vi "Teleop.vi"(10 "Match Info":T1={"Autonomous Elapsed Seconds"=0.0, "TeleOp Elapsed Seconds"=0.0, "Disabled Elapsed Seconds"=0.0, "Visited Autonomous"=FALSE, "Visited TeleOp"=FALSE, "Visited Disabled"=FALSE, "Autonomous Settings"={"Autonomous Style"=enum."Independent", "VI Refnum"=refnum}}, 11 "Call Context":T2) -> ()   [LabVIEW 2016]
doc: "This VI is called for each TeleOp packet received from the DS where the robot is not disabled. It is often used to read from the joysticks and update I/O or to update setpoints for timed control loops. It should complete and return within 20 milliseconds or it may miss DS packets."
uses:
  <vilib>/Rock Robotics/WPI/DriverStation/WPI_DriverStationDerivedRobotMode.ctl
  <vilib>/Rock Robotics/WPI/DriverStation/WPI_DriverStationMatch Info.ctl
  <vilib>/Rock Robotics/WPI/Relay/WPI_RelayValue.ctl
  <vilib>/Rock Robotics/WPI/Solenoid/WPI_SolenoidValue.ctl
  <vilib>/Rock Robotics/WPI/ThirdParty/CanMotor/TalonSRX/WPI_CANTalonSRX_BrakeOverride.ctl
  <vilib>/Rock Robotics/WPI/Utilities/WPI_GetSetVariantRefNum.vi
  <vilib>/Rock Robotics/Network Tables/NT Write Boolean Array.vi
  <vilib>/Rock Robotics/Network Tables/NT Write Numeric Array.vi
  <vilib>/Rock Robotics/Network Tables/NT Read Boolean.vi
  <vilib>/Rock Robotics/Network Tables/NT Read Number.vi
  <vilib>/Rock Robotics/Network Tables/NT Write Boolean.vi
  <vilib>/addons/control/pid/pid.llb/PID (DBL).vi
  <vilib>/Rock Robotics/WPI/Solenoid/WPI_SolenoidSetEnum.vi
  <vilib>/Rock Robotics/WPI/RobotDrive/WPI_RobotDriveArcadeDrive_Standard(NoSaturation).vi
  <vilib>/addons/control/pid/NI_PID_pid.lvlib
panel:
  out "percentRateLeft":dbl
  out "percentRateRight":dbl
  out "motorOutputInit":dbl
  out "motorOutputInit":dbl
  out "encRateLeft":dbl
  out "encRateRight":dbl
  out "outputLeft":dbl format="%.2f"
  out "outputRight":dbl format="%.2f"
  out "Sample Slider 0":dbl(slide) scale=0.0..5.0
  out "Sample Boolean 1":bool
  out "Sample Boolean 0":bool
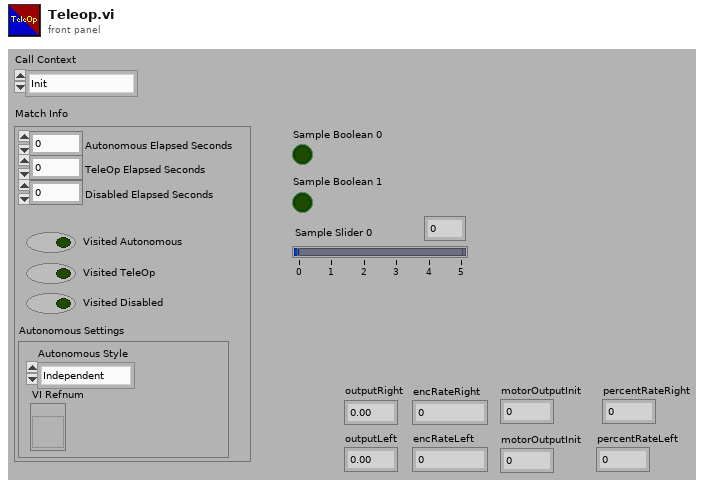
[diagram p1: front panel]
types:
  T1 = typedef "WPI_DriverStationMatch Info.ctl" = cluster{"Autonomous Elapsed Seconds":dbl, "TeleOp Elapsed Seconds":dbl, "Disabled Elapsed Seconds":dbl, "Visited Autonomous":bool, "Visited TeleOp":bool, "Visited Disabled":bool, "Autonomous Settings":cluster{"Autonomous Style":enum16{"Iterative", "Independent"}, "VI Refnum":refnum<vi>}}
  T2 = typedef "WPI_DriverStationDerivedRobotMode.ctl" = enum16{"Init", "Execute", "Stop"}
  T3 = cluster{"proportional gain (Kc)":dbl, "integral time (Ti, min)":dbl, "derivative time (Td, min)":dbl}
  T4 = typedef "WPI_CANTalonSRX_BrakeOverride.ctl" = enum8{"No Override", "Override to Coast", "Override to Brake"}
  T5 = typedef "WPI_SolenoidValue.ctl" = enum16{"Off", "On", "Forward", "Reverse"}
  T6 = typedef "WPI_RelayValue.ctl" = enum16{"Off", "On", "Forward", "Reverse"}
  T7 = typedef "WPI_JoystickDevRef.ctl" = cluster{"Device":T8}
  T8 = typedef "WPI_JoystickDeviceEnum.ctl" = enum16{"USB 0", "USB 1", "USB 2", "USB 3", "USB 4", "USB 5"}
  T9 = typedef "WPI_RobotDriveDevRef.ctl" = cluster{"DevStatus":errorcluster, "Motors[]":T10[], "Square Inputs":bool, "Max Output":dbl}
  T10 = typedef "WPI_MotorControlDeviceRef.ctl" = cluster{"DeviceStatus":errorcluster, "Type":T11, "PWM":cluster{"PWM Channel":T12, "DeadBand":T13}, "CAN":cluster{"Device Number":u8, "SetOutput VI Ref":variant, "GetOutput VI Ref":variant, "Enable VI Ref":variant, "Disable VI Ref":variant, "Data":variant}, "Invert":bool}
  T11 = typedef "WPI_MotorControlType.ctl" = enum16{"PWM", "CAN"}
  T12 = typedef "FPGA_DIOPWMChannel.ctl" = enum8{"PWM 0", "PWM 1", "PWM 2", "PWM 3", "PWM 4", "PWM 5", "PWM 6", "PWM 7", "PWM 8", "PWM 9", "PWM MXP 0", "PWM MXP 1", "PWM MXP 2", "PWM MXP 3", "PWM MXP 4", "PWM MXP 5", "PWM MXP 6", "PWM MXP 7", "PWM MXP 8", "PWM MXP 9", "Invalid"}
  T13 = typedef "WPI_PWMDeadband.ctl" = cluster{"Name":string, "maxPositivePwm":i32, "minPositivePwm":i32, "centerPwm":i32, "maxNegativePwm":i32, "minNegativePwm":i32, "angularRange":u16}
  T14 = typedef "WPI_RelayDevRef.ctl" = cluster{"DevStatus":errorcluster, "Relay Channel":T15, "Relay Direction":T16}
  T15 = typedef "FPGA_DIORelayChannel.ctl" = enum8{"Relay 0", "Relay 1", "Relay 2", "Relay 3", "Invalid"}
  T16 = typedef "WPI_RelayDirection.ctl" = enum16{"Both directions", "Forward only", "Reverse only"}
  T17 = typedef "WPI_SolenoidDevRef.ctl" = cluster{"DevStatus":errorcluster, "Pneumatics Control Module":u8, "Forward Solenoid Channel":T18, "Reverse Solenoid Channel":T18}
  T18 = typedef "WPI_SolenoidChannel.ctl" = enum8{"Solenoid 0", "Solenoid 1", "Solenoid 2", "Solenoid 3", "Solenoid 4", "Solenoid 5", "Solenoid 6", "Solenoid 7", "Invalid"}
  T19 = typedef "WPI_EncoderDevRef.ctl" = cluster{"DevStatus":errorcluster, "EncoderIndex":T20, "CounterIndex":T21, "DistancePerCount":dbl, "Decoding Type":T22}
  T20 = typedef "FPGA_EncoderIdx.ctl" = enum8{"Enc 0", "Enc 1", "Enc 2", "Enc 3", "Enc 4", "Enc 5", "Enc 6", "Enc 7", "Invalid"}
  T21 = typedef "FPGA_CounterCtrSystemIndex.ctl" = enum8{"Ctr 0", "Ctr 1", "Ctr 2", "Ctr 3", "Ctr 4", "Ctr 5", "Ctr 6", "Ctr 7", "Invalid"}
  T22 = typedef "WPI_EncoderType.ctl" = enum16{"1x", "2x", "4x"}
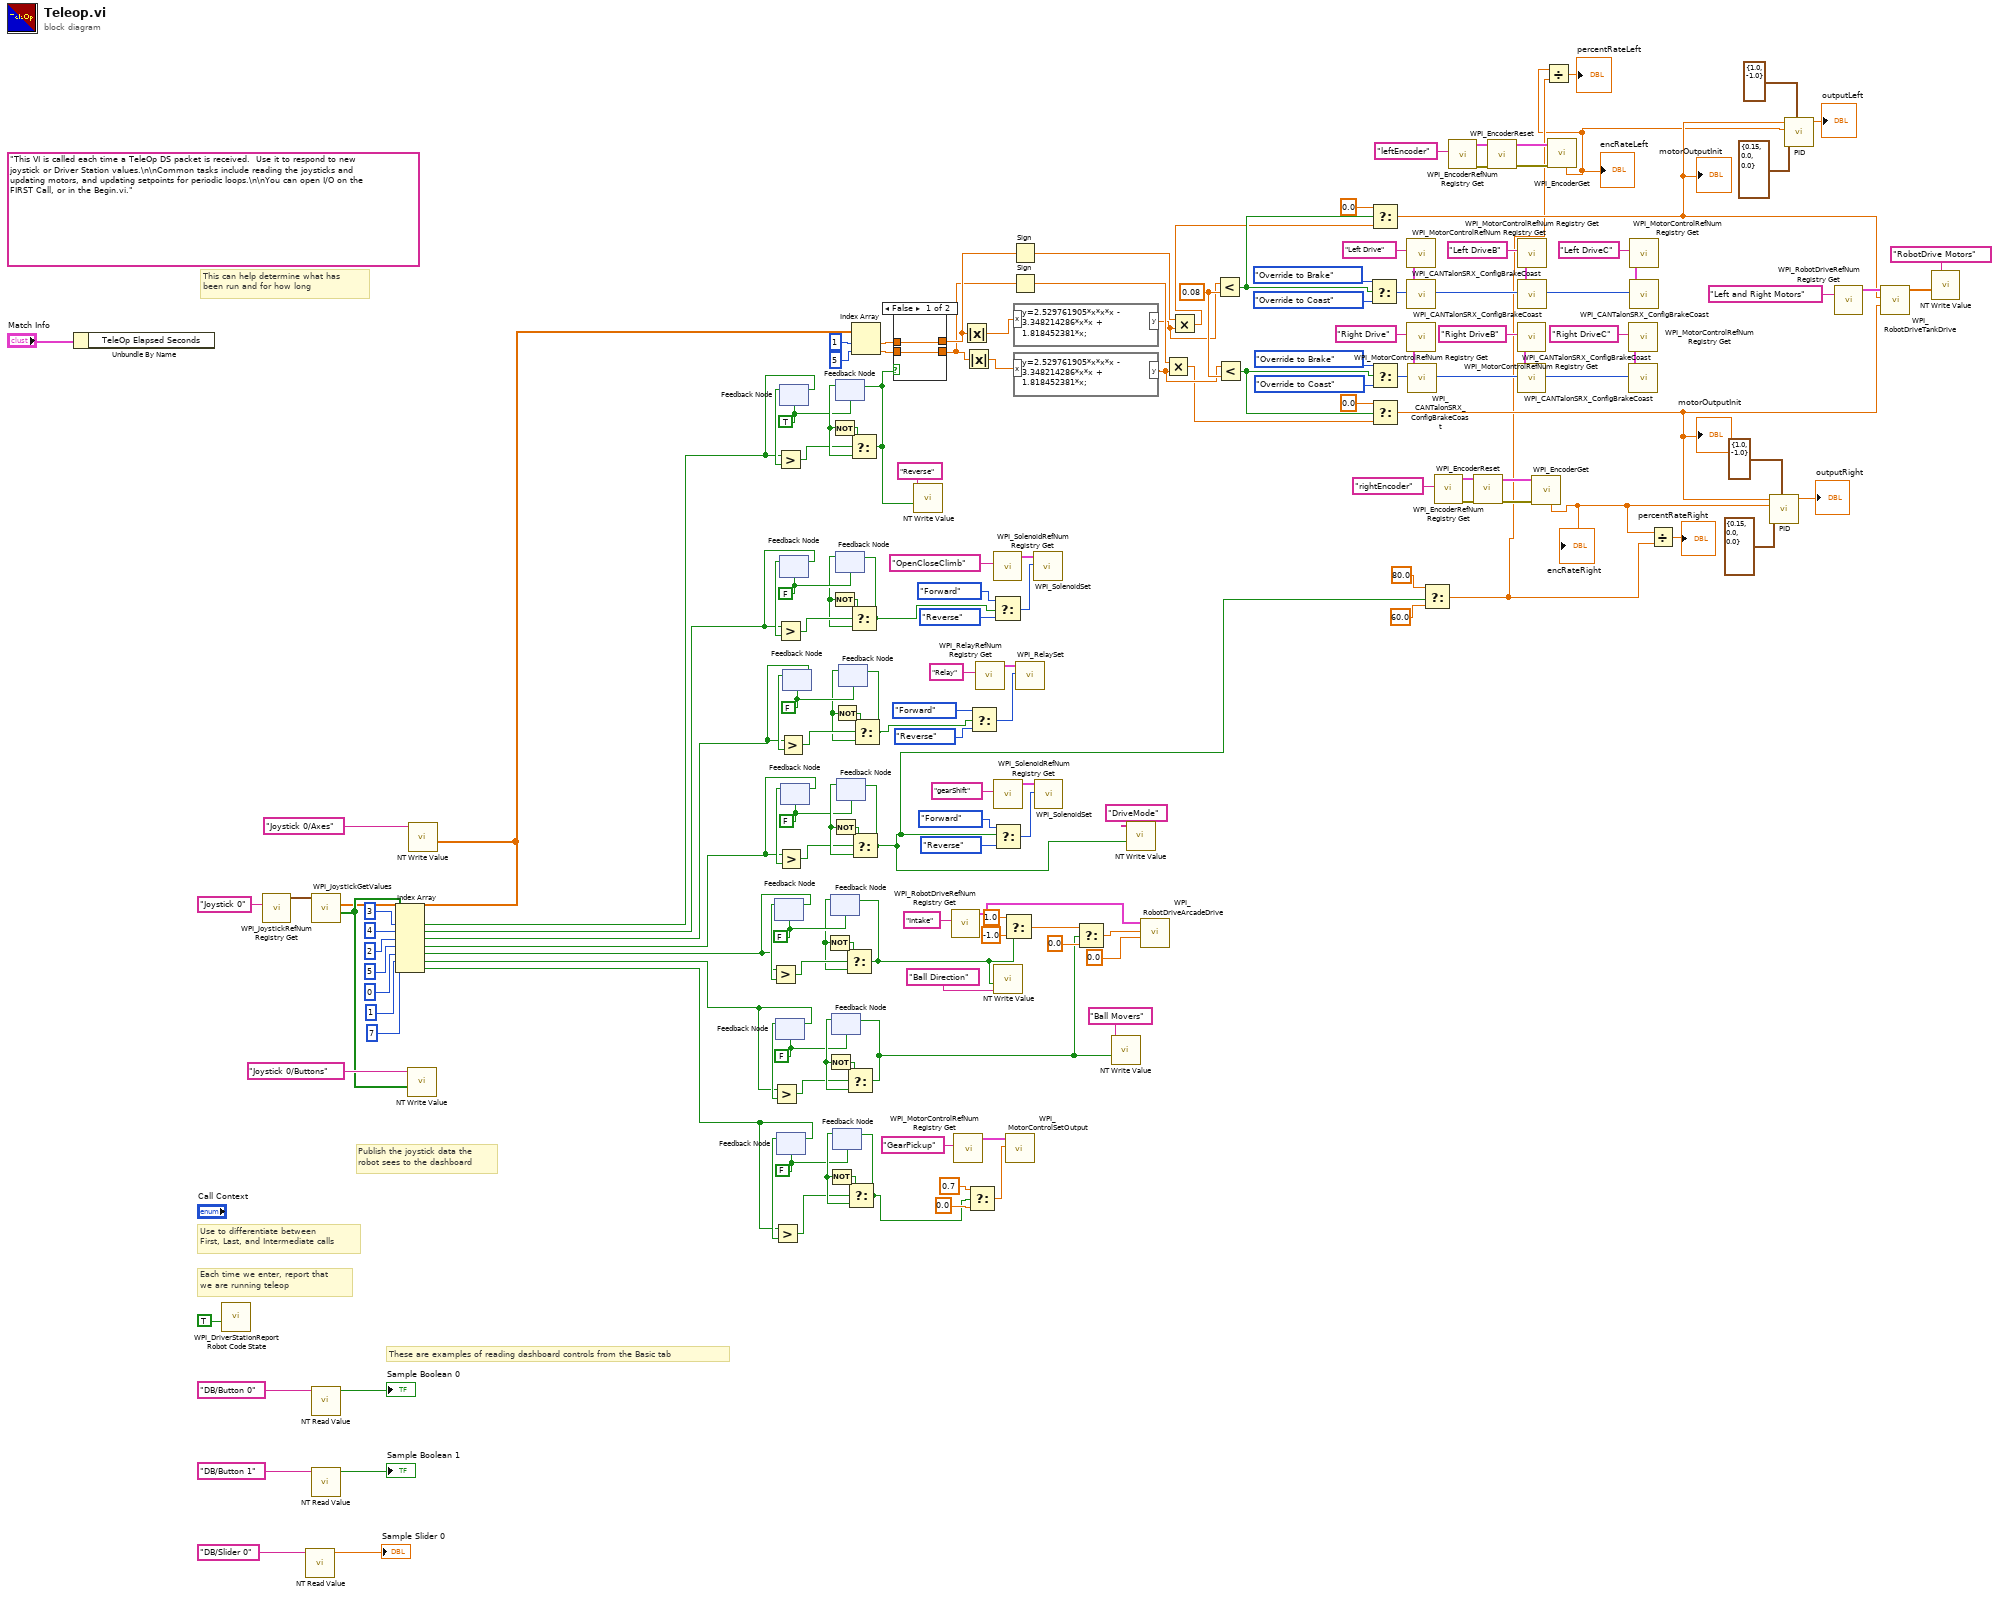
[diagram p0: block diagram]
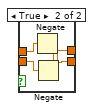
[diagram p2: hidden frame]
diagram:
  w45 = 0.08 ("y")
  w73 = TRUE ("Boolean")
  w102 = FALSE ("Boolean")
  w128 = FALSE ("Boolean")
  w133 = FALSE ("Boolean")
  w138 = FALSE ("Boolean")
  w143 = FALSE ("Boolean")
  w148 = FALSE ("Boolean")
  (unwired) "This VI is called each time a TeleOp DS packet is received.  Use it to respond to new joystick or Driver Station values.\n\nCommon tasks include reading the joysticks and updating motors, and updating setpoints for periodic loops.\n\nYou can open I/O on the FIRST Call, or in the Begin.vi."
  # "These are examples of reading dashboard controls from the Basic tab"
  # "Publish the joystick data the\nrobot sees to the dashboard"
  # "Each time we enter, report that\nwe are running teleop"
  # "Use to differentiate between\nFirst, Last, and Intermediate calls"
  # "This can help determine what has\nbeen run and for how long"
  n1 = Unbundle By Name("Match Info") -> ()  [unwired: 1 out]
  n2 = call <vilib>:"WPI_DriverStationReport Robot Code State.vi"("TeleOp"=TRUE ("Autonomous")) -> ()  [unwired: 10 in, 1 out]
  n3 = call <vilib>:"WPI_JoystickRefNum Registry Get.vi"("refnum name"="Joystick 0") -> ("JoystickDevRef"=w166:T7)  [unwired: 1 in, 9 out]
  n4 = call-poly <vilib>:"NT Read Value.vi"("Name"="DB/Slider 0" ("refnum name")) -> ("Numeric"=→"Sample Slider 0":dbl)  [unwired: 9 in, 1 out]
  n5 = call <vilib>:"WPI_JoystickGetValues.vi"("JoystickDevRef"=w166) -> ("Buttons"=w156:bool[], "Axes"=w67:dbl[])  [unwired: 6 in, 3 out]
  n6 = call-poly <vilib>:"NT Read Value.vi"("Name"="DB/Button 0" ("refnum name")) -> ("Boolean"=→"Sample Boolean 0":bool)  [unwired: 9 in, 1 out]
  n7 = call-poly <vilib>:"NT Read Value.vi"("Name"="DB/Button 1" ("refnum name")) -> ("Boolean"=→"Sample Boolean 1":bool)  [unwired: 9 in, 1 out]
  n8 = Index Array(array=w156, index #1=3 ("index"), index #2=4 ("index"), index #3=2 ("index"), index #4=5 ("index"), index #5=0 ("index"), index #6=1 ("index"), index #7=7 ("index")) -> (element #1=w66:bool, element #2=w65:bool, element #3=w64:bool, element #4=w63:bool, element #5=w62:bool, element #6=w61:bool, element #7=w60:bool)
  n9 = call-poly <vilib>:"NT Write Value.vi"("Boolean Array"=w156, "Name"="Joystick 0/Buttons") -> ()  [unwired: 9 in, 1 out]
  n10 = call-poly <vilib>:"NT Write Value.vi"("Numeric Array"=w67, "Name"="Joystick 0/Axes") -> ()  [unwired: 9 in, 1 out]
  n11 = feedback #1(w133) -> (w135:bool)
  n12 = Greater?(x=w62, y=w135) -> (0:w134:bool)
  n13 = feedback-in #1(w62) -> ()
  n14 = feedback #2(w102) -> (w100:bool)
  n15 = Greater?(x=w61, y=w100) -> (0:w101:bool)
  n16 = feedback-in #2(w61) -> ()
  n17 = feedback #3(w128) -> (w126:bool)
  n18 = Greater?(x=w60, y=w126) -> (0:w127:bool)
  n19 = feedback-in #3(w60) -> ()
  n20 = feedback #4(w73) -> (w71:bool)
  n21 = Greater?(x=w66, y=w71) -> (0:w72:bool)
  n22 = feedback-in #4(w66) -> ()
  n23 = feedback #5(w148) -> (w150:bool)
  n24 = Greater?(x=w65, y=w150) -> (0:w149:bool)
  n25 = feedback-in #5(w65) -> ()
  n26 = feedback #6(w138) -> (w136:bool)
  n27 = Greater?(x=w63, y=w136) -> (0:w137:bool)
  n28 = feedback-in #6(w63) -> ()
  n29 = feedback #7(w143) -> (w145:bool)
  n30 = Greater?(x=w64, y=w145) -> (0:w144:bool)
  n31 = feedback-in #7(w64) -> ()
  n32 = feedback #8(w133) -> (w132:bool)
  n33 = Not(x=w132) -> (.not. x?=w131:bool)
  n34 = feedback #9(w102) -> (w103:bool)
  n35 = Not(x=w103) -> (.not. x?=w104:bool)
  n36 = feedback #10(w128) -> (w129:bool)
  n37 = Not(x=w129) -> (.not. x?=w130:bool)
  n38 = feedback #11(w73) -> (w74:bool)
  n39 = Not(x=w74) -> (.not. x?=w75:bool)
  n40 = feedback #12(w148) -> (w147:bool)
  n41 = Not(x=w147) -> (.not. x?=w146:bool)
  n42 = feedback #13(w138) -> (w139:bool)
  n43 = Not(x=w139) -> (.not. x?=w140:bool)
  n44 = feedback #14(w143) -> (w142:bool)
  n45 = Not(x=w142) -> (.not. x?=w141:bool)
  n46 = Select(t=w131, s=w134, f=w132) -> (s? t:f=w84:bool)
  n47 = feedback-in #8(w84) -> ()
  n48 = Select(t=w104, s=w101, f=w103) -> (s? t:f=w85:bool)
  n49 = feedback-in #9(w85) -> ()
  n50 = Select(t=w130, s=w127, f=w129) -> (s? t:f=w89:bool)
  n51 = feedback-in #10(w89) -> ()
  n52 = Select(t=w75, s=w72, f=w74) -> (s? t:f=w69:bool)
  n53 = feedback-in #11(w69) -> ()
  n54 = Select(t=w146, s=w149, f=w147) -> (s? t:f=w125:bool)
  n55 = feedback-in #12(w125) -> ()
  n56 = Select(t=w140, s=w137, f=w139) -> (s? t:f=w6:bool)
  n57 = feedback-in #13(w6) -> ()
  n58 = Index Array(array=w67, index #1=1 ("index"), index #2=5 ("index")) -> (element #1=w77:dbl, element #2=w76:dbl)
  n59 = Select(t=w141, s=w144, f=w142) -> (s? t:f=w114:bool)
  n60 = feedback-in #14(w114) -> ()
  n61 = case shown="False" w69 {
    tunnel: [w170 w172] -> w57
    tunnel: w77 -> [w170 w174]
    tunnel: [w169 w171] -> w56
    tunnel: w76 -> [w169 w173]
    frame False {
    }
    frame True {
      n62 = Negate(x=w174) -> (-x=w171:dbl)
      n63 = Negate(x=w173) -> (-x=w172:dbl)
    }
  }
  n64 = call-poly <vilib>:"NT Write Value.vi"("Boolean"=w69, "Name"="Reverse") -> ()  [unwired: 9 in, 1 out]
  n65 = call <vilib>:"WPI_RobotDriveRefNum Registry Get.vi"("refnum name"="Intake") -> ("RobotDriveDevRef"=w94:T9)  [unwired: 9 in, 1 out]
  n66 = call <vilib>:"WPI_MotorControlRefNum Registry Get.vi"("refnum name"="GearPickup") -> ("MotorControlDevRef"=w88:T10)  [unwired: 9 in, 1 out]
  n67 = Absolute Value(x=w57) -> (abs(x)=w59:dbl)
  n68 = Absolute Value(x=w56) -> (abs(x)=w58:dbl)
  n69 = Select(t=0.7, s=w89, f=0.0 ("Output")) -> (s? t:f=w90:dbl)
  n70 = Select(t=WPI_RelayValue."Forward" ("RelayValue"), s=w114, f=WPI_RelayValue."Reverse") -> (s? t:f=w117:T6)
  n71 = call <vilib>:"WPI_RelayRefNum Registry Get.vi"("refnum name"="Relay") -> ("RelayDevRef"=w118:T14)  [unwired: 9 in, 1 out]
  n72 = call <vilib>:"WPI_SolenoidRefNum Registry Get.vi"("refnum name"="OpenCloseClimb") -> ("SolenoidDevRef"=w121:T17)  [unwired: 9 in, 1 out]
  n73 = Select(t=WPI_SolenoidValue."Forward" ("Value"), s=w125, f=WPI_SolenoidValue."Reverse" ("Value")) -> (s? t:f=w120:T5)
  n74 = call <vilib>:"WPI_SolenoidRefNum Registry Get.vi"("refnum name"="gearShift") -> ("SolenoidDevRef"=w109:T17)  [unwired: 9 in, 1 out]
  n75 = Select(t=WPI_SolenoidValue."Forward" ("Value"), s=w6, f=WPI_SolenoidValue."Reverse" ("Value")) -> (s? t:f=w111:T5)
  n76 = call-poly <vilib>:"NT Write Value.vi"("Boolean"=w84, "Name"="Ball Direction") -> ()  [unwired: 9 in, 1 out]
  n77 = Select(t=1.0, s=w84, f=-1.0) -> (s? t:f=w98:dbl)
  n78 = call <vilib>:"WPI_MotorControlSetOutput.vi"("Output"=w90, "MotorControlDevRef"=w88) -> ()  [unwired: 7 in, 3 out]
  n79 = Sign(1:w57) -> (0:w54:dbl)
  n80 = Sign(1:w56) -> (0:w55:dbl)
  n81 = formula code="y=2.529761905*x*x*x - 3.348214286*x*x + 1.818452381*x;"("x"=w59) -> ("y"=w40:dbl)
  n82 = formula code="y=2.529761905*x*x*x - 3.348214286*x*x + 1.818452381*x;"("x"=w58) -> ("y"=w38:dbl)
  n83 = call <vilib>:"WPI_RelaySet.vi"("RelayValue"=w117, "RelayDevRef"=w118) -> ()  [unwired: 8 in, 2 out]
  n84 = call-poly <vilib>:"WPI_SolenoidSet.vi"("Value"=w120, "SolenoidDevRef"=w121) -> ()  [unwired: 8 in, 2 out]
  n85 = call-poly <vilib>:"WPI_SolenoidSet.vi"("Value"=w111, "SolenoidDevRef"=w109) -> ()  [unwired: 8 in, 2 out]
  n86 = Select(t=w98, s=w85, f=0.0) -> (s? t:f=w97:dbl)
  n87 = call-poly <vilib>:"NT Write Value.vi"("Boolean"=w85, "Name"="Ball Movers") -> ()  [unwired: 9 in, 1 out]
  n88 = call-poly <vilib>:"NT Write Value.vi"("Boolean"=w6, "Name"="DriveMode") -> ()  [unwired: 9 in, 1 out]
  n89 = call-poly <vilib>:"WPI_RobotDriveArcadeDrive.vi"("Y axis value"=0.0, "X axis value"=w97, "RobotDriveDevRef"=w94) -> ()  [unwired: 6 in, 3 out]
  n90 = Multiply(x=w55, y=w38) -> (x*y=w37:dbl)
  n91 = Multiply(x=w54, y=w40) -> (x*y=w39:dbl)
  n92 = Less?(x=w40, y=w45) -> (x < y?=w43:bool)
  n93 = Less?(x=w38, y=w45) -> (x < y?=w44:bool)
  n94 = Select(t=WPI_CANTalonSRX_BrakeOverride."Override to Brake" ("Brake / Coast Mode"), s=w43, f=WPI_CANTalonSRX_BrakeOverride."Override to Coast") -> (s? t:f=w27:T4)
  n95 = Select(t=0.0, s=w43, f=w39) -> (s? t:f=w12:dbl)
  "motorOutputInit" <- w12
  n96 = Select(t=WPI_CANTalonSRX_BrakeOverride."Override to Brake" ("Brake / Coast Mode"), s=w44, f=WPI_CANTalonSRX_BrakeOverride."Override to Coast") -> (s? t:f=w32:T4)
  n97 = Select(t=0.0, s=w44, f=w37) -> (s? t:f=w11:dbl)
  "motorOutputInit" <- w11
  n98 = call <vilib>:"WPI_MotorControlRefNum Registry Get.vi"("refnum name"="Left Drive") -> ("MotorControlDevRef"=w46:T10)  [unwired: 9 in, 1 out]
  n99 = call <vilib>:"WPI_CANTalonSRX_ConfigBrakeCoast.vi"("Brake / Coast Mode"=w27, "CAN Talon SRX Ref"=w46) -> ()  [unwired: 8 in, 2 out]
  n100 = call <vilib>:"WPI_MotorControlRefNum Registry Get.vi"("refnum name"="Right Drive") -> ("MotorControlDevRef"=w49:T10)  [unwired: 9 in, 1 out]
  n101 = call <vilib>:"WPI_CANTalonSRX_ConfigBrakeCoast.vi"("Brake / Coast Mode"=w32, "CAN Talon SRX Ref"=w49) -> ()  [unwired: 8 in, 2 out]
  n102 = Select(t=80.0, s=w6, f=60.0) -> (s? t:f=w2:dbl)
  n103 = call <vilib>:"WPI_EncoderRefNum Registry Get.vi"("refnum name"="rightEncoder") -> ("error out"=w22:errorcluster, "EncoderDevRef"=w23:T19)  [unwired: 9 in]
  n104 = call <vilib>:"WPI_EncoderRefNum Registry Get.vi"("refnum name"="leftEncoder") -> ("error out"=w16:errorcluster, "EncoderDevRef"=w15:T19)  [unwired: 9 in]
  n105 = call <vilib>:"WPI_EncoderReset.vi"("error in (no error)"=w22, "EncoderDevRef"=w23) -> ("error out"=w20:errorcluster, "EncoderDevRef"=w21:T19)  [unwired: 8 in]
  n106 = call <vilib>:"WPI_EncoderReset.vi"("error in (no error)"=w16, "EncoderDevRef"=w15) -> ("error out"=w13:errorcluster, "EncoderDevRef"=w14:T19)  [unwired: 8 in]
  n107 = call <vilib>:"WPI_MotorControlRefNum Registry Get.vi"("refnum name"="Right DriveB") -> ("MotorControlDevRef"=w35:T10)  [unwired: 9 in, 1 out]
  n108 = call <vilib>:"WPI_CANTalonSRX_ConfigBrakeCoast.vi"("Brake / Coast Mode"=w32, "CAN Talon SRX Ref"=w35) -> ()  [unwired: 8 in, 2 out]
  n109 = call <vilib>:"WPI_MotorControlRefNum Registry Get.vi"("refnum name"="Left DriveB") -> ("MotorControlDevRef"=w30:T10)  [unwired: 9 in, 1 out]
  n110 = call <vilib>:"WPI_CANTalonSRX_ConfigBrakeCoast.vi"("Brake / Coast Mode"=w27, "CAN Talon SRX Ref"=w30) -> ()  [unwired: 8 in, 2 out]
  n111 = call <vilib>:"WPI_EncoderGet.vi"("error in (no error)"=w20, "EncoderDevRef"=w21) -> ("Rate"=w5:dbl)  [unwired: 4 in, 5 out]
  "encRateRight" <- w5
  n112 = call <vilib>:"WPI_EncoderGet.vi"("error in (no error)"=w13, "EncoderDevRef"=w14) -> ("Rate"=w1:dbl)  [unwired: 4 in, 5 out]
  "encRateLeft" <- w1
  n113 = Divide(x=w1, y=w2) -> (x/y=→"percentRateLeft":dbl)
  n114 = call <vilib>:"WPI_MotorControlRefNum Registry Get.vi"("refnum name"="Right DriveC") -> ("MotorControlDevRef"=w33:T10)  [unwired: 9 in, 1 out]
  n115 = call <vilib>:"WPI_CANTalonSRX_ConfigBrakeCoast.vi"("Brake / Coast Mode"=w32, "CAN Talon SRX Ref"=w33) -> ()  [unwired: 8 in, 2 out]
  n116 = call <vilib>:"WPI_MotorControlRefNum Registry Get.vi"("refnum name"="Left DriveC") -> ("MotorControlDevRef"=w28:T10)  [unwired: 9 in, 1 out]
  n117 = call <vilib>:"WPI_CANTalonSRX_ConfigBrakeCoast.vi"("Brake / Coast Mode"=w27, "CAN Talon SRX Ref"=w28) -> ()  [unwired: 8 in, 2 out]
  n118 = Divide(x=w5, y=w2) -> (x/y=→"percentRateRight":dbl)
  n119 = call-poly <vilib>:"PID.vi"("output range"=cluster{"output high":dbl, "output low":dbl} {"output high"=1.0, "output low"=-1.0}, "PID gains"=T3 {"proportional gain (Kc)"=0.15, "integral time (Ti, min)"=0.0, "derivative time (Td, min)"=0.0}, "process variable"=w5, "setpoint"=w11) -> ("output"=→"outputRight":dbl)  [unwired: 6 in, 1 out]
  n120 = call-poly <vilib>:"PID.vi"("output range"=cluster{"output high":dbl, "output low":dbl} {"output high"=1.0, "output low"=-1.0}, "PID gains"=T3 {"proportional gain (Kc)"=0.15, "integral time (Ti, min)"=0.0, "derivative time (Td, min)"=0.0}, "process variable"=w1, "setpoint"=w12) -> ("output"=→"outputLeft":dbl)  [unwired: 6 in, 1 out]
  n121 = call <vilib>:"WPI_RobotDriveRefNum Registry Get.vi"("refnum name"="Left and Right Motors") -> ("RobotDriveDevRef"=w82:T9)  [unwired: 1 in, 9 out]
  n122 = call <vilib>:"WPI_RobotDriveTankDrive.vi"("Right axis value"=w11, "Left axis value"=w12, "RobotDriveDevRef"=w82) -> ("Motor Values"=w81:dbl[])  [unwired: 6 in, 2 out]
  n123 = call-poly <vilib>:"NT Write Value.vi"("Numeric Array"=w81, "Name"="RobotDrive Motors") -> ()  [unwired: 9 in, 1 out]
